vi "get_IVRP_waveform.vi"(10 "Channel config":T2={"Voltage channel index"=1, "Shunt channel index"=2, "Shunt resistance"=10.0}, 11 "array":waveform(dbl)[](array[waveform])) -> (0 "Voltage waveform out":waveform(dbl), 1 "Power waveform out":waveform(dbl), 2 "Resistance waveform out":waveform(dbl), 3 "Current waveform out":waveform(dbl), 4 "Channel names":T1)   [LabVIEW 2020]
doc: "This example demonstrates how to acquire a continuous amount of data (Waveform) using the DAQ device's internal clock. It also shows how to synchronize two devices for different device families (E Series, S Series, M Series, X Series, DSA, and SC Express), to simultaneously acquire the data.\n\nFor instructions on how to connect your signals to the DAQ device, refer to your device documentation."
panel:
  # "Get IVRP Waveform"
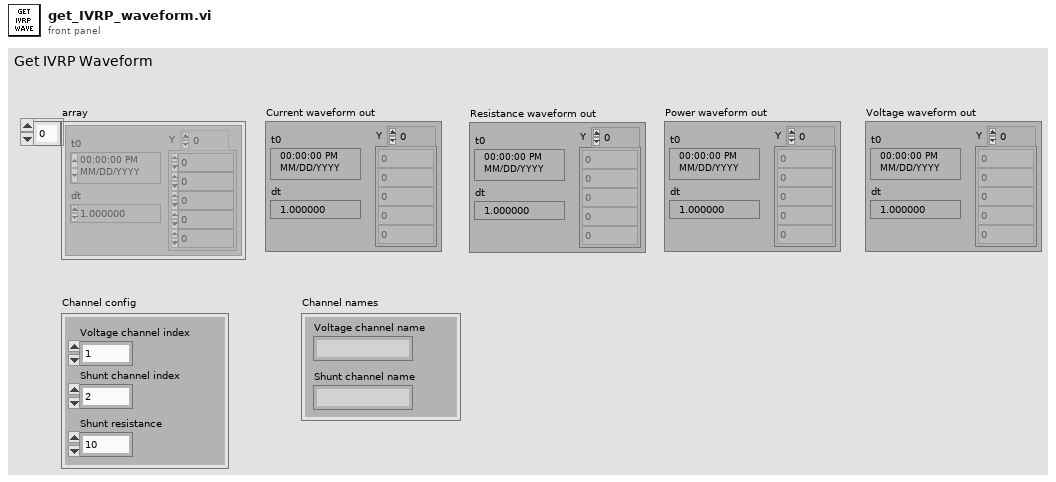
[diagram p1: front panel]
types:
  T1 = cluster{"Voltage channel name":string, "Shunt channel name":string}
  T2 = cluster{"Voltage channel index":i32, "Shunt channel index":i32, "Shunt resistance":dbl}
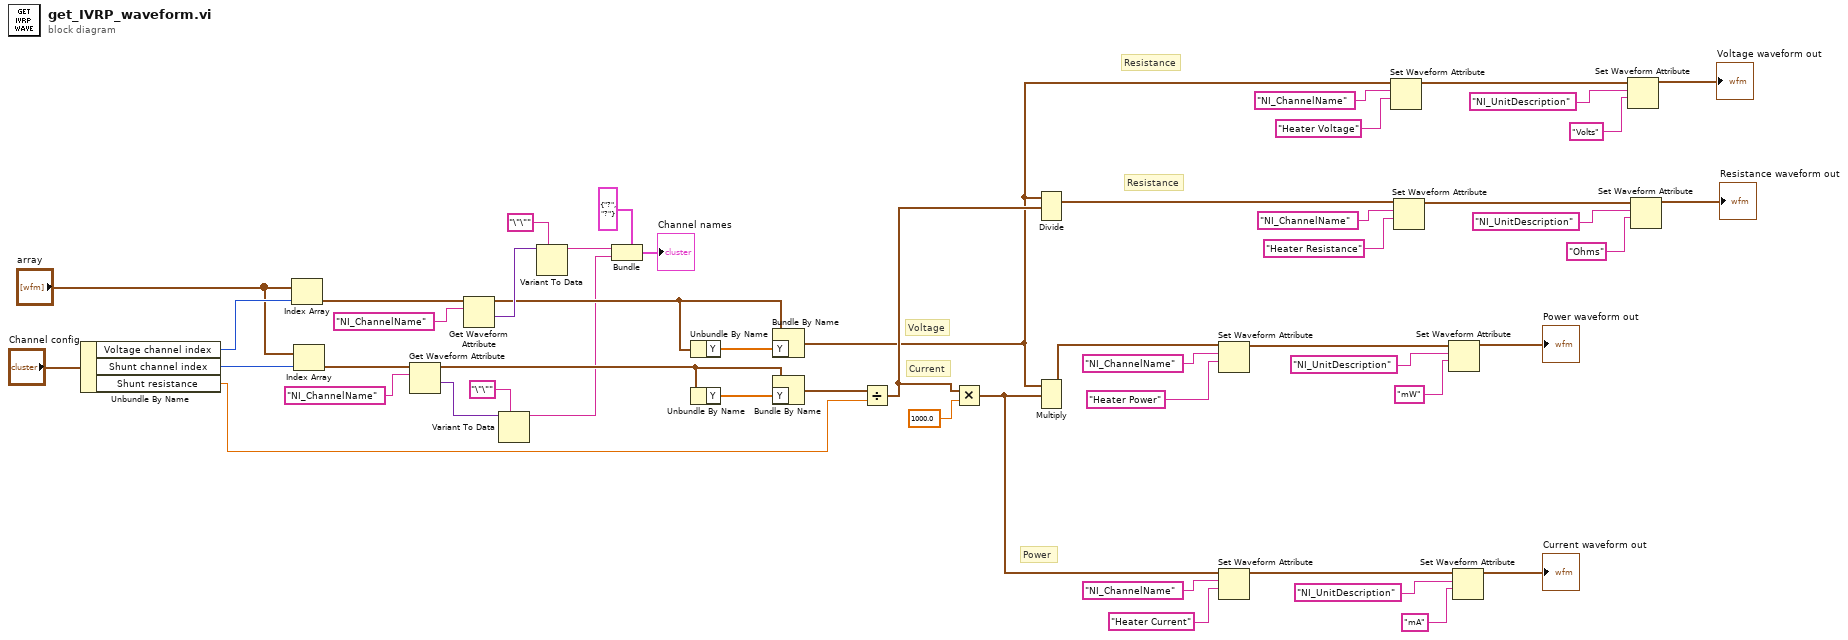
[diagram p0: block diagram]
diagram:
  # "Resistance"
  # "Power"
  # "Resistance"
  # "Voltage"
  # "Current"
  n1 = Unbundle By Name("Channel config") -> ("Voltage channel index"=w44:i32, "Shunt channel index"=w38:i32, "Shunt resistance"=w8:dbl)
  n2 = Index Array(array="array", index=w44) -> (element=w48:waveform(dbl))
  n3 = Index Array(array="array", index=w38) -> (element=w33:waveform(dbl))
  n4 = Get Waveform Attribute(6:"NI_ChannelName" ("name"), 7:w33) -> (1:w34:variant, 3:w31:waveform(dbl))  [unwired: 2 in, 2 out]
  n5 = Get Waveform Attribute(6:"NI_ChannelName" ("name"), 7:w48) -> (1:w42:variant, 3:w41:waveform(dbl))  [unwired: 2 in, 2 out]
  n6 = Variant To Data(type="\"\"" ("name"), Variant=w34) -> (data=w13:string)  [unwired: 1 in, 1 out]
  n7 = Variant To Data(type="\"\"" ("name"), Variant=w42) -> (data=w14:string)  [unwired: 1 in, 1 out]
  n8 = Bundle(cluster=cluster{"name":string, "name":string} {"name"="?", "name"="?"}, "name"=w14, "name"=w13) -> (→"Channel names":cluster{"name":string, "name":string})
  n9 = Unbundle By Name(w41) -> ("Y"=w40:dbl[])
  n10 = Unbundle By Name(w31) -> ("Y"=w32:dbl[])
  n11 = Bundle By Name(cluster=w41, "Y"=w40) -> (w1:waveform(dbl))
  n12 = Bundle By Name(cluster=w31, "Y"=w32) -> (w16:waveform(dbl))
  n13 = Divide(x=w16, y=w8) -> (x/y=w9:waveform(dbl))
  n14 = Multiply(x=w9, y=1000.0) -> (x*y=w10:waveform(dbl))
  n15 = Divide(1:w9, 2:w1) -> (0:w15:waveform(dbl))  [unwired: 1 in, 1 out]
  n16 = Multiply(1:w10, 2:w1) -> (0:w39:waveform(dbl))  [unwired: 1 in, 1 out]
  n17 = Set Waveform Attribute(5:"Heater Power" ("name"), 6:"NI_ChannelName" ("name"), 7:w39) -> (3:w50:waveform(dbl))  [unwired: 1 in, 2 out]
  n18 = Set Waveform Attribute(5:"Heater Current" ("name"), 6:"NI_ChannelName" ("name"), 7:w10) -> (3:w23:waveform(dbl))  [unwired: 1 in, 2 out]
  n19 = Set Waveform Attribute(5:"Heater Voltage" ("name"), 6:"NI_ChannelName" ("name"), 7:w1) -> (3:w5:waveform(dbl))  [unwired: 1 in, 2 out]
  n20 = Set Waveform Attribute(5:"Heater Resistance" ("name"), 6:"NI_ChannelName" ("name"), 7:w15) -> (3:w28:waveform(dbl))  [unwired: 1 in, 2 out]
  n21 = Set Waveform Attribute(5:"mW" ("name"), 6:"NI_UnitDescription" ("name"), 7:w50) -> (3:→"Power waveform out":waveform(dbl))  [unwired: 1 in, 2 out]
  n22 = Set Waveform Attribute(5:"mA" ("name"), 6:"NI_UnitDescription" ("name"), 7:w23) -> (3:→"Current waveform out":waveform(dbl))  [unwired: 1 in, 2 out]
  n23 = Set Waveform Attribute(5:"Volts" ("name"), 6:"NI_UnitDescription" ("name"), 7:w5) -> (3:→"Voltage waveform out":waveform(dbl))  [unwired: 1 in, 2 out]
  n24 = Set Waveform Attribute(5:"Ohms" ("name"), 6:"NI_UnitDescription" ("name"), 7:w28) -> (3:→"Resistance waveform out":waveform(dbl))  [unwired: 1 in, 2 out]
